vi "Configure Edge Time.vi"(4 "Upper Reference Value (90%)":dbl=90.0 format="%#_4g", 6 "Lower Reference Value (10%)":dbl=10.0 format="%#_4g", 8 "error in (no error)":errorcluster, 9 "Reference Type (0:Percent)":i32(ring) items=["Percent", "Volts"], 10 "Edge Time Type (0:Rise)":i32(ring) items=["Rise", "Fall"], 11 "VISA resource name":refnum<visa-resource-name>) -> (0 "error out":errorcluster, 3 "VISA resource name out":refnum<visa-resource-name>)   [LabVIEW 2020, in "Counter.lvlib" / "PICOTEST U62XXA series.lvlib"]
doc: "Configures Edge Time measurements. Edge Time measurements can only be taken at channel 1.\n\n<B>Note:</B>\n\nThe U6220A model <B>does not</B> support the \"Edge Time\" commands."
uses:
  PICOTEST U62XXA series.lvlib
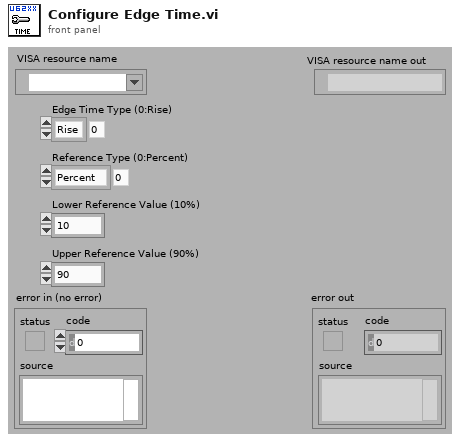
[diagram p1: front panel]
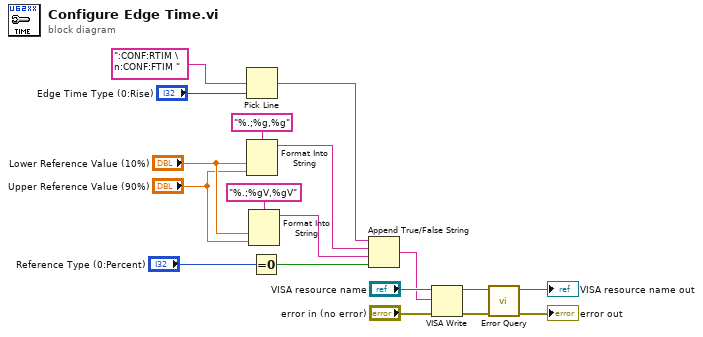
[diagram p0: block diagram]
diagram:
  n1 = Pick Line(multi-line string=":CONF:RTIM \n:CONF:FTIM ", line index="Edge Time Type (0:Rise)") -> (output string=w1:string)  [unwired: 1 in]
  n2 = Format Into String(format string="%.;%g,%g", "Lower Reference Value (10%)", "Upper Reference Value (90%)") -> (resulting string=w3:string)  [unwired: 2 in, 1 out]
  n3 = Format Into String(format string="%.;%gV,%gV", "Lower Reference Value (10%)", "Upper Reference Value (90%)") -> (resulting string=w2:string)  [unwired: 2 in, 1 out]
  n4 = Equal To 0?(x="Reference Type (0:Percent)") -> (x = 0?=w14:bool)
  n5 = Append True/False String(1:w14, 2:w2, 3:w3, 4:w1) -> (0:w13:string)
  n6 = VISA Write(VISA resource name="VISA resource name", write buffer=w13, error in (no error)="error in (no error)") -> (VISA resource name out=w12:refnum<visa-resource-name>, error out=w10:errorcluster)  [unwired: 1 out]
  n7 = call "Error Query.vi"("error in (no error)"=w10, "VISA resource name"=w12) -> ("error out"=→"error out":errorcluster, "VISA resource name out"=→"VISA resource name out":refnum<visa-resource-name>)  [unwired: 6 in, 2 out]
